vi "Close Down.vi"(10 "error in (no error)":errorcluster, 11 "FPGA Interface":refnum<k20>) -> (0 "error out":errorcluster)   [LabVIEW 2016]
doc: "Inputs\nFPGA reference\n\nOutputs\n-\n\nThis VI shuts down the forward and steering motor, deactivates the walkassist mode and activates the brake motor. It also turn off the communcation LED and stops the FPGA."
uses:
  <vilib>/Utility/error.llb/Error Cluster From Error Code.vi
  <vilib>/rvi/errors/niLvFpgaAdjustHostInterfaceError.vi
  <vilib>/FPGAPlugInAG/Dynamic/niLvFpga_Abort_Dynamic.vi
  <vilib>/FPGAPlugInAG/Dynamic/niLvFpga_Close_Dynamic.vi
  <vilib>/rvi/interface/nirviReadWriteControl/nirviReadWriteControl.xnode
  <vilib>/rvi/interface/nirviMethod/nirviMethod.xnode
  <vilib>/rvi/interface/nirviCloseFPGA/nirviCloseFPGA.xnode
  NiFpgaLv.dll
  <vilib>/rvi/interface/Simulation/niFpgaSimulationCallBeginRW.vi
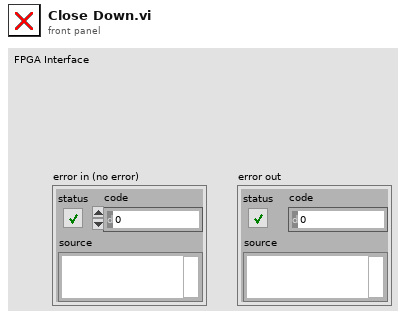
[diagram p1: front panel]
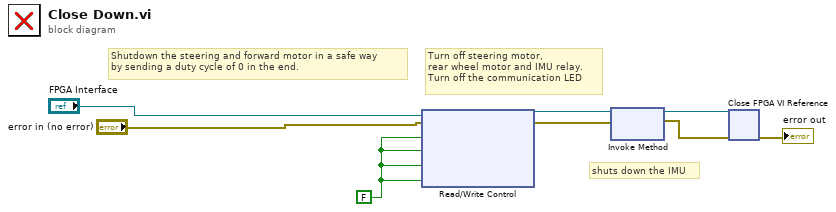
[diagram p0: block diagram]
diagram:
  w1 = FALSE
  # "shuts down the IMU"
  # "Turn off steering motor,\nrear wheel motor and IMU relay.\nTurn off the communication LED"
  # "Shutdown the steering and forward motor in a safe way \nby sending a duty cycle of 0 in the end."
  n1 = xnode "Read/Write Control"("FPGA VI Reference In"="FPGA Interface", "error in"="error in (no error)", "MotorsON"=w1, "Comm LED Red"=w1, "IMU ON?"=w1, "Comm LED Green"=w1) -> ("FPGA VI Reference Out"=w5:refnum<k20>, "error out"=w4:errorcluster)
  n2 = xnode "Invoke Method"("FPGA VI Reference In"=w5, "error in"=w4) -> ("FPGA VI Reference Out"=w7:refnum<k20>, "error out"=w6:errorcluster)
  n3 = xnode "Close FPGA VI Reference"("FPGA VI Reference In"=w7, "error in"=w6) -> ("error out"=→"error out":errorcluster)
